vi "Set_Visible.vi"(8 "error in (no error)":errorcluster, 9 "Visible?":bool=TRUE, 10 "Control Label":string, 11 "CtlLookup In":T1) -> (0 "error out":errorcluster, 3 "CtlLookup Out":T1)   [LabVIEW 2020, in "CtlReferences.lvlib" / "CtlReferences.lvclass"]
doc: "Toggles visibility of specified control"
uses:
  CtlReferences.lvclass
  TypeDefs/CtlLookup.ctl
  Error_CtlNotFound.vi
  <vilib>/Utility/error.llb/Error Cluster From Error Code.vi
  Error_ToSpecificClass.vi
  CtlReferences.lvclass/CtlReferences.ctl
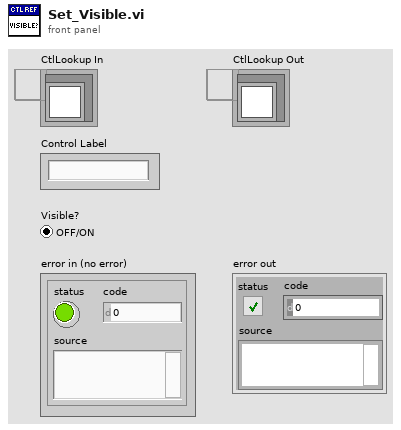
[diagram p1: front panel]
types:
  T1 = typedef "CtlReferences.lvlib/CtlReferences.lvclass/CtlLookup.ctl" = refnum<data-value>
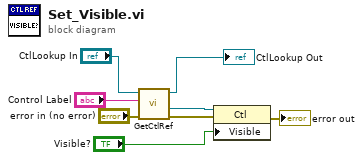
[diagram p0: block diagram]
diagram:
  n1 = call "GetCtlRef.vi"("Error in"="error in (no error)", "CtlName In"="Control Label", "CtlLookup In"="CtlLookup In") -> ("error out"=w6:errorcluster, "CtlRef"=w5:refnum<vi>, "CtlLookup Out"=→"CtlLookup Out":T1)  [unwired: 5 in, 1 out]
  n2 = property class="Ctl"(reference=w5, error in=w6, "Visible"="Visible?") -> (error out=→"error out":errorcluster)  [unwired: 1 out]
